vi "LVClass_WavefrontCorrector Get Actuator Preferences.vi"(0 "WavefrontCorrector in":refnum<class "WavefrontCorrector.lvclass">, 5 "Index of actuator":i32, 11 "error in (no error)":errorcluster) -> (4 "WavefrontCorrector out":refnum<class "WavefrontCorrector.lvclass">, 6 "Wavefront Corrector State":T1, 15 "error out":errorcluster)   [LabVIEW 2020, in "WavefrontCorrector.lvclass"]
uses:
  WavefrontCorrector.lvclass
  Wavefront Corrector states - ONE.ctl
  WavefrontCorrector.lvclass/WavefrontCorrector.ctl
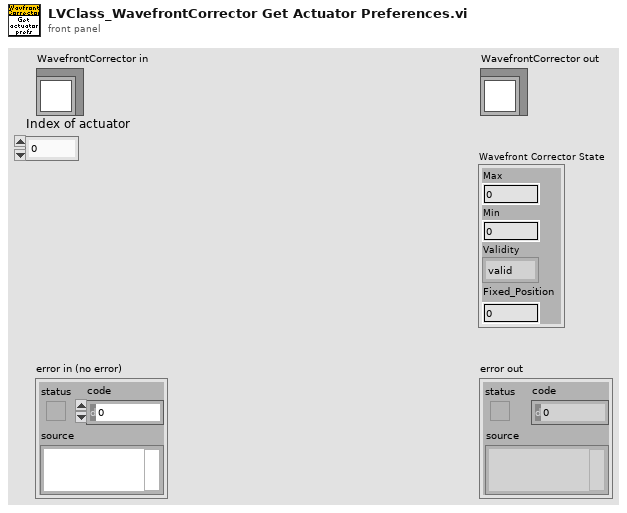
[diagram p1: front panel]
types:
  T1 = typedef "Wavefront Corrector states - ONE.ctl" = cluster{"Max":sgl, "Min":sgl, "Validity":enum16{"valid", "fixed", "invalid"}, "Fixed_Position":sgl}
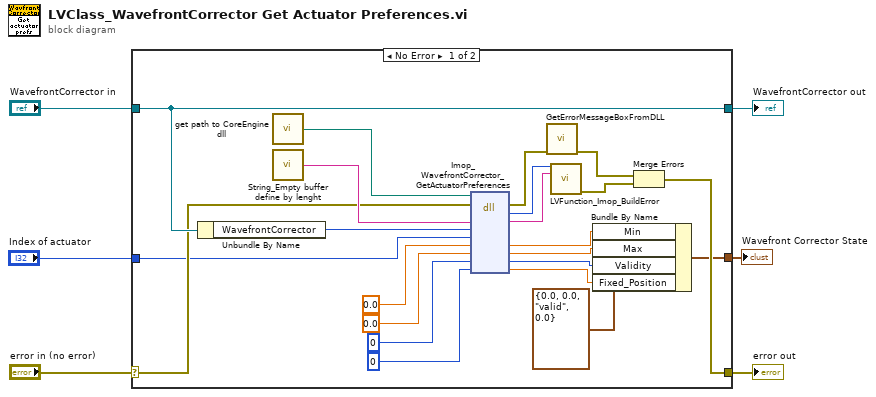
[diagram p0: block diagram]
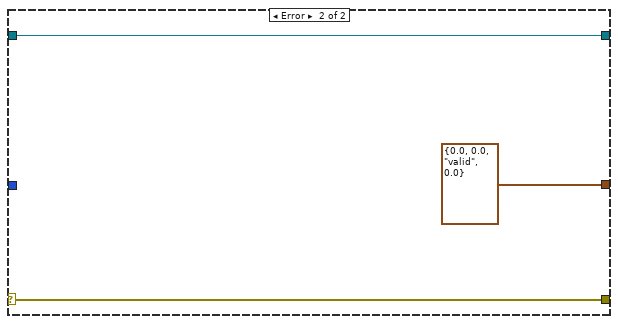
[diagram p2: hidden frame]
diagram:
  n1 = case shown="No Error" "error in (no error)" {
    selector: "error in (no error)" -> [w15 w31]
    tunnel: [w14 w31] -> w5
    tunnel: [w26 w30] -> w3
    tunnel: "WavefrontCorrector in" -> [w26 w30]
    tunnel: [w8 T1 {"Max"=0.0, "Min"=0.0, "Validity"=enum."valid", "Fixed_Position"=0.0} ("Actuator state")] -> w2
    tunnel: "Index of actuator" -> [w7 _]
    frame No Error {
      n2 = Unbundle By Name(w26) -> ("WavefrontCorrector"=w25:i32)
      n3 = call "get path to CoreEngine dll.vi"() -> ("path to c_interface_vc100.dll"=w28:path)  [unwired: 12 in, 3 out]
      n4 = call "String_Empty buffer define by lenght.vi"() -> ("Empty buffer"=w27:string)  [unwired: 1 in]
      n5 = dll-call lib="D:/FLE/0.Code/CoreEngine4_Suite/LV2011_interface/DLLs/c_interface_vc100.dll" fn="Imop_WavefrontCorrector_GetActuatorPreferences"(path in=w28, error in=w15, "Message"=w27, "Wavefront Corrector"=w25, "Index of actuator"=w7, "Min"=sgl 0.0, "Max"=sgl 0.0, "Validity"=0, "Fixed_positions"=0) -> (error out=w20:errorcluster, "return type"=w18:i32, "Message"=w17:string, "Min"=w12:sgl, "Max"=w11:sgl, "Validity"=w10:i32, "Fixed_positions"=w9:sgl)  [unwired: 3 in, 1 out]
      n6 = call "GetErrorMessageBoxFromDLL.vi"("error IN"=w20) -> ("error OUT"=w19:errorcluster)  [unwired: 10 in]
      n7 = call "LVFunction_Imop_BuildError.vi"("code"=w18, "String to Prepend to source (\"\")"=w17) -> ("error out"=w16:errorcluster)  [unwired: 13 in]
      n8 = Bundle By Name(cluster=T1 {"Max"=0.0, "Min"=0.0, "Validity"=enum."valid", "Fixed_Position"=0.0} ("Actuator state"), "Min"=w12, "Max"=w11, "Validity"=w10, "Fixed_Position"=w9) -> (w8:T1)
      n9 = Merge Errors(w19, w16) -> (w14:errorcluster)
    }
    frame Error {
    }
  }
  "error out" <- w5
  "WavefrontCorrector out" <- w3
  "Wavefront Corrector State" <- w2
